vi "Merge.vi"(6 "Conditional Object":refnum<class>, 8 "error in (no error)":errorcluster, 9 "Object B":refnum<class>, 10 "Object A":refnum<class>, 11 "Overwrite A if default in":refnum<class "Overwrite A if is default.lvclass">) -> (0 "error out":errorcluster, 2 "Output Object":refnum<class>, 3 "Overwrite A if default out":refnum<class "Overwrite A if is default.lvclass">)   [LabVIEW 2020, in "Merge Tools.lvlib" / "Overwrite A if is default.lvclass"]
uses:
  Overwrite A if is default.lvclass
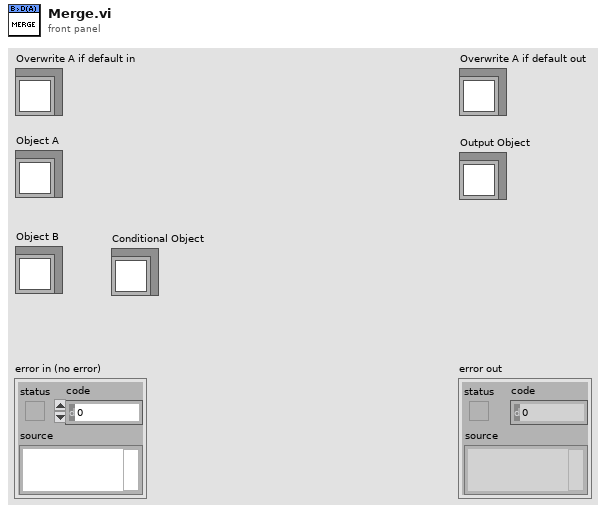
[diagram p1: front panel]
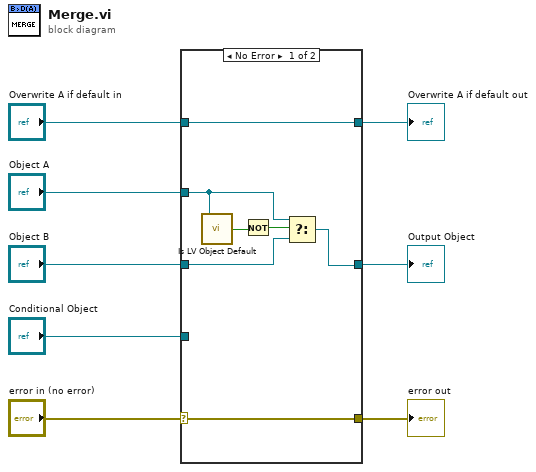
[diagram p0: block diagram]
diagram:
  n1 = case shown="No Error" "error in (no error)" {
    selector: "error in (no error)" -> [w15 w17]
    tunnel: [w15 w17] -> w7
    tunnel: "Overwrite A if default in" -> [w14 w16]
    tunnel: [w14 w16] -> w5
    tunnel: "Object A" -> [w11 _]
    tunnel: "Object B" -> [w10 _]
    tunnel: "Conditional Object" -> [_ _]
    tunnel: [w9 _] -> w1
    frame No Error {
      n2 = call "Is LV Object Default.vi"("LabVIEW Object"=w11) -> ("Is Default?"=w13:bool)
      n3 = Not(x=w13) -> (.not. x?=w12:bool)
      n4 = Select(t=w11, s=w12, f=w10) -> (s? t:f=w9:refnum<class>)
    }
    frame Error {
    }
  }
  "error out" <- w7
  "Overwrite A if default out" <- w5
  "Output Object" <- w1
